vi "_dump_or_value.vi"(8 "error in (no error)":errorcluster, 10 "indent":T1, 11 "value":refnum<class "Node.lvclass">) -> (0 "error out":errorcluster, 2 "mlir":string)   [LabVIEW 2020, in "mlir.lvlib"]
uses:
  mlir.lvlib
  Node/Node.lvclass
  Node/indent.ctl
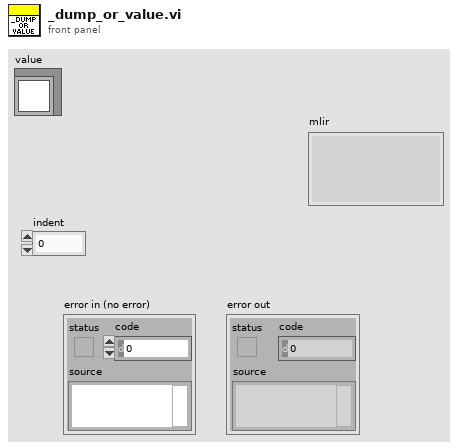
[diagram p1: front panel]
types:
  T1 = typedef "mlir.lvlib/indent.ctl" = u32
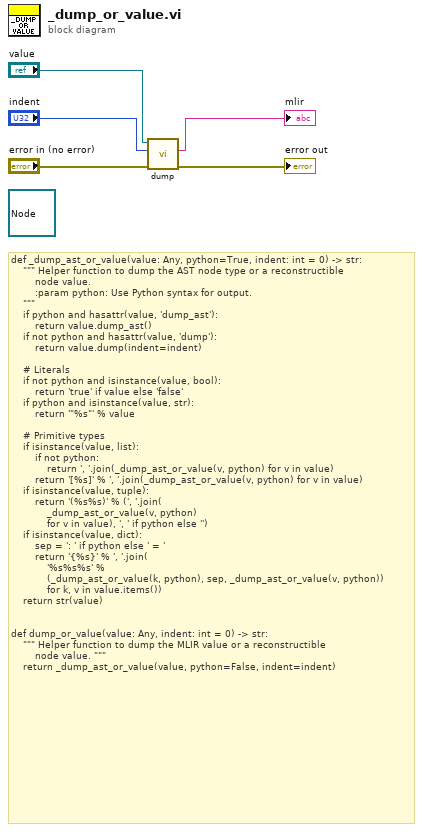
[diagram p0: block diagram]
diagram:
  (unwired) refnum<class "Node.lvclass"> refnum ("mlir.lvlib:Node.lvclass")
  # "def _dump_ast_or_value(value: Any, python=True, indent: int = 0) -> str:\n    \"\"\" Helper function to dump the AST node type or a reconstructible\n        node value.\n        :param python: Use Python syntax for output.\n    \"\"\"\n    if python and hasattr(value, 'dump_ast'):\n        return value.dump_ast()\n    if not python and hasattr(value, 'dump'):\n        return value.dump(indent=indent)\n\n    # Literals\n    if not python and isinstance(value, bool):\n        return 'true' if value else 'false'\n    if python and isinstance(value, str):\n        return '\"%s\"' % value\n\n    # Primitive types\n    if isinstance(value, list):\n        if not python:\n            return ', '.join(_dump_ast_or_value(v, python) for v in value)\n        return '[%s]' % ', '.join(_dump_ast_or_value(v, python) for v in value)\n    if isinstance(value, tuple):\n        return '(%s%s)' % (', '.join(\n            _dump_ast_or_value(v, python)\n            for v in value), ', ' if python else '')\n    if isinstance(value, dict):\n        sep = ': ' if python else ' = '\n        return '{%s}' % ', '.join(\n            '%s%s%s' %\n            (_dump_ast_or_value(k, python), sep, _dump_ast_or_value(v, python))\n            for k, v in value.items())\n    return str(value)\n\n\ndef dump_or_value(value: Any, indent: int = 0) -> str:\n    \"\"\" Helper function to dump the MLIR value or a reconstructible\n        node value. \"\"\"\n    return _dump_ast_or_value(value, python=False, indent=indent)"
  n1 = call-dynamic "dump.vi"("error in (no error)"="error in (no error)", "indent"="indent", "Node in"="value") -> ("error out"=→"error out":errorcluster, "mlir"=→"mlir":string)  [unwired: 6 in, 1 out]
